vi "Superimpose_Anomaly_Map.vi"(5 "Gamma":i32, 7 "Alpha":sgl, 10 "Anomaly Map":u32[][](array[numeric]), 11 "Image":u32[][](array[numeric])) -> (3 "Img out":u32[][](array[numeric]))   [LabVIEW 2020]
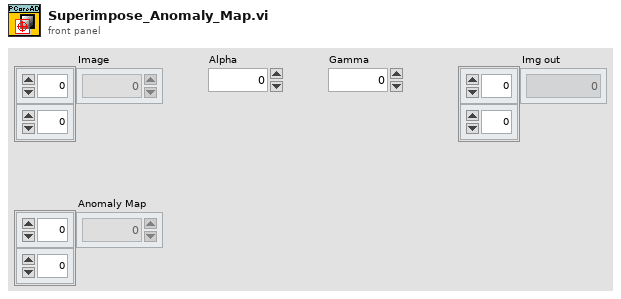
[diagram p1: front panel]
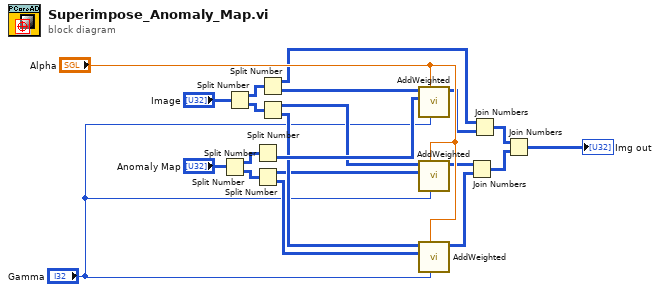
[diagram p0: block diagram]
diagram:
  n1 = Split Number(x="Anomaly Map") -> (hi(x)=w20:u16[][], lo(x)=w21:u16[][])
  n2 = Split Number(x="Image") -> (hi(x)=w18:u16[][], lo(x)=w19:u16[][])
  n3 = Split Number(x=w20) -> (lo(x)=w14:u8[][])  [unwired: 1 out]
  n4 = Split Number(x=w21) -> (hi(x)=w8:u8[][], lo(x)=w11:u8[][])
  n5 = Split Number(x=w18) -> (hi(x)=w1:u8[][], lo(x)=w15:u8[][])
  n6 = Split Number(x=w19) -> (hi(x)=w13:u8[][], lo(x)=w12:u8[][])
  n7 = call "AddWeighted.vi"("Gamma"="Gamma", "Alpha"="Alpha", "Src2"=w14, "Src1"=w15) -> ("Weighted Add"=w7:u8[][])  [unwired: 7 in]
  n8 = call "AddWeighted.vi"("Gamma"="Gamma", "Alpha"="Alpha", "Src2"=w8, "Src1"=w13) -> ("Weighted Add"=w6:u8[][])  [unwired: 7 in]
  n9 = call "AddWeighted.vi"("Gamma"="Gamma", "Alpha"="Alpha", "Src2"=w11, "Src1"=w12) -> ("Weighted Add"=w5:u8[][])  [unwired: 7 in]
  n10 = Join Numbers(hi=w6, lo=w5) -> ((hi.lo)=w4:u16[][])
  n11 = Join Numbers(hi=w1, lo=w7) -> ((hi.lo)=w3:u16[][])
  n12 = Join Numbers(hi=w3, lo=w4) -> ((hi.lo)=→"Img out":u32[][])
